vi "clusster.vi"() -> ()   [LabVIEW 2020]
panel:
  out "XY Graph":cluster{"X":dbl, "Y":dbl}[](graph)
  out "cluster":T1
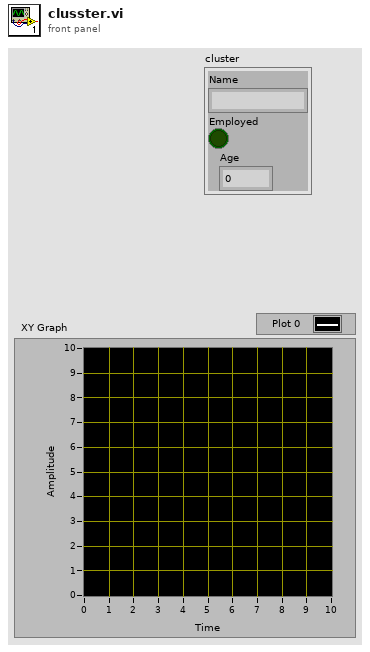
[diagram p1: front panel]
types:
  T1 = cluster{"Name":string, "Employed":bool, "Age":dbl}
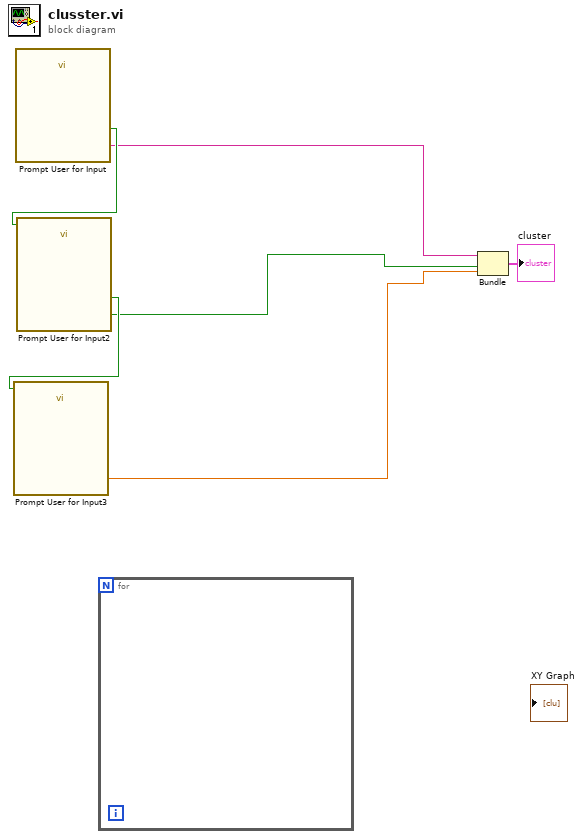
[diagram p0: block diagram]
diagram:
  n1 = call "Prompt User for Input"() -> ("Name"=w1:string, "OK"=w6:bool)  [unwired: 17 in, 1 out]
  n2 = call "Prompt User for Input2"("Enable"=w6) -> ("Employed"=w2:bool, "OK"=w5:bool)  [unwired: 16 in, 1 out]
  n3 = call "Prompt User for Input3"("Enable"=w5) -> ("Age"=w3:dbl)  [unwired: 16 in, 2 out]
  n4 = for {
  }
  n5 = Bundle("Name"=w1, "Employed"=w2, "Age"=w3) -> (→"cluster":T1)  [unwired: 1 in]
